vi "Get Resource.vi"(8 "error in (no error)":errorcluster, 11 "Device in":refnum<class "Device.lvclass">) -> (0 "error out":errorcluster, 2 "Resource":refnum<class "DeployResource.lvclass">, 3 "Device out":refnum<class "Device.lvclass">)   [LabVIEW 2020, in "PicoG-Core.lvlib" / "Device.lvclass"]
uses:
  Device.lvclass
  DeployResource/DeployResource.lvclass
  Device.lvclass/Device.ctl
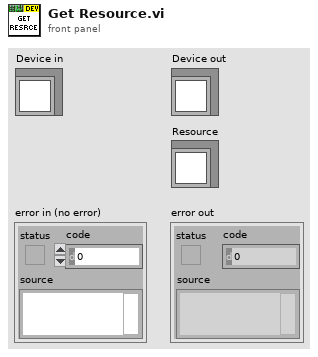
[diagram p1: front panel]
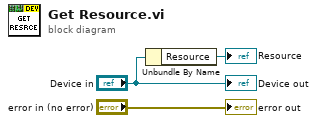
[diagram p0: block diagram]
diagram:
  n1 = Unbundle By Name("Device in") -> ("Resource"=→"Resource":refnum<class "DeployResource.lvclass">)
  "error out" <- "error in (no error)"
  "Device out" <- "Device in"
